vi "test_Series cRIO PWM TC Temp.vi"(8 "Error In":errorcluster) -> (0 "Error Out":errorcluster)   [LabVIEW 2023]
uses:
  DIO/DO DAQmx Fixed Freq PWM CFG/DO DAQmx Fixed Freq PWM CFG.lvclass
  Devices/NEO480HTA/Real All CFG/Read All CFG.lvclass
  Series/Series Base/Series Base.lvclass
  <vilib>/ActorFramework/Actor/Actor.lvclass
  <vilib>/ActorFramework/Stop Msg/Stop Msg.lvclass
  Sample Tasks/Sample Airtemp PWM Control/Sample Airtemp PWM Control.lvclass
  Thermometer/Virtual Thermometers/Virt Temperature Reader/Virt Temperature Reader.lvclass
  Series/Series Actor/Series Actor/Series Actor.lvclass
  Series/ISeries Actor/ISeries Actor Messages/Start Tasks Msg/Start Tasks Msg.lvclass
  Series/ISeries Actor/ISeries Actor Messages/Stop Tasks Msg/Stop Tasks Msg.lvclass
  DIO/Virtual DIO/Virt PWM Fixed Freq Generator/Virt DAQmx Fixed Freq PWM Generator.lvclass
panel:
  out "Aircooler Dutycycle":dbl=23.0
  in  "Start Series Button":bool
  in  "Kill Series Actor Button":bool
  out "Temperature Chart Lossy":dbl(graph)
  in  "Temp Setpoint":dbl=23.0 format="%#_g °C"
  in  "stop":bool
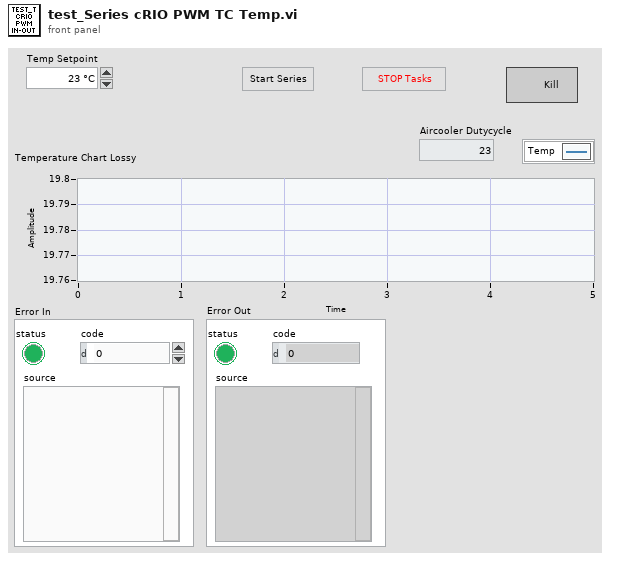
[diagram p1: front panel]
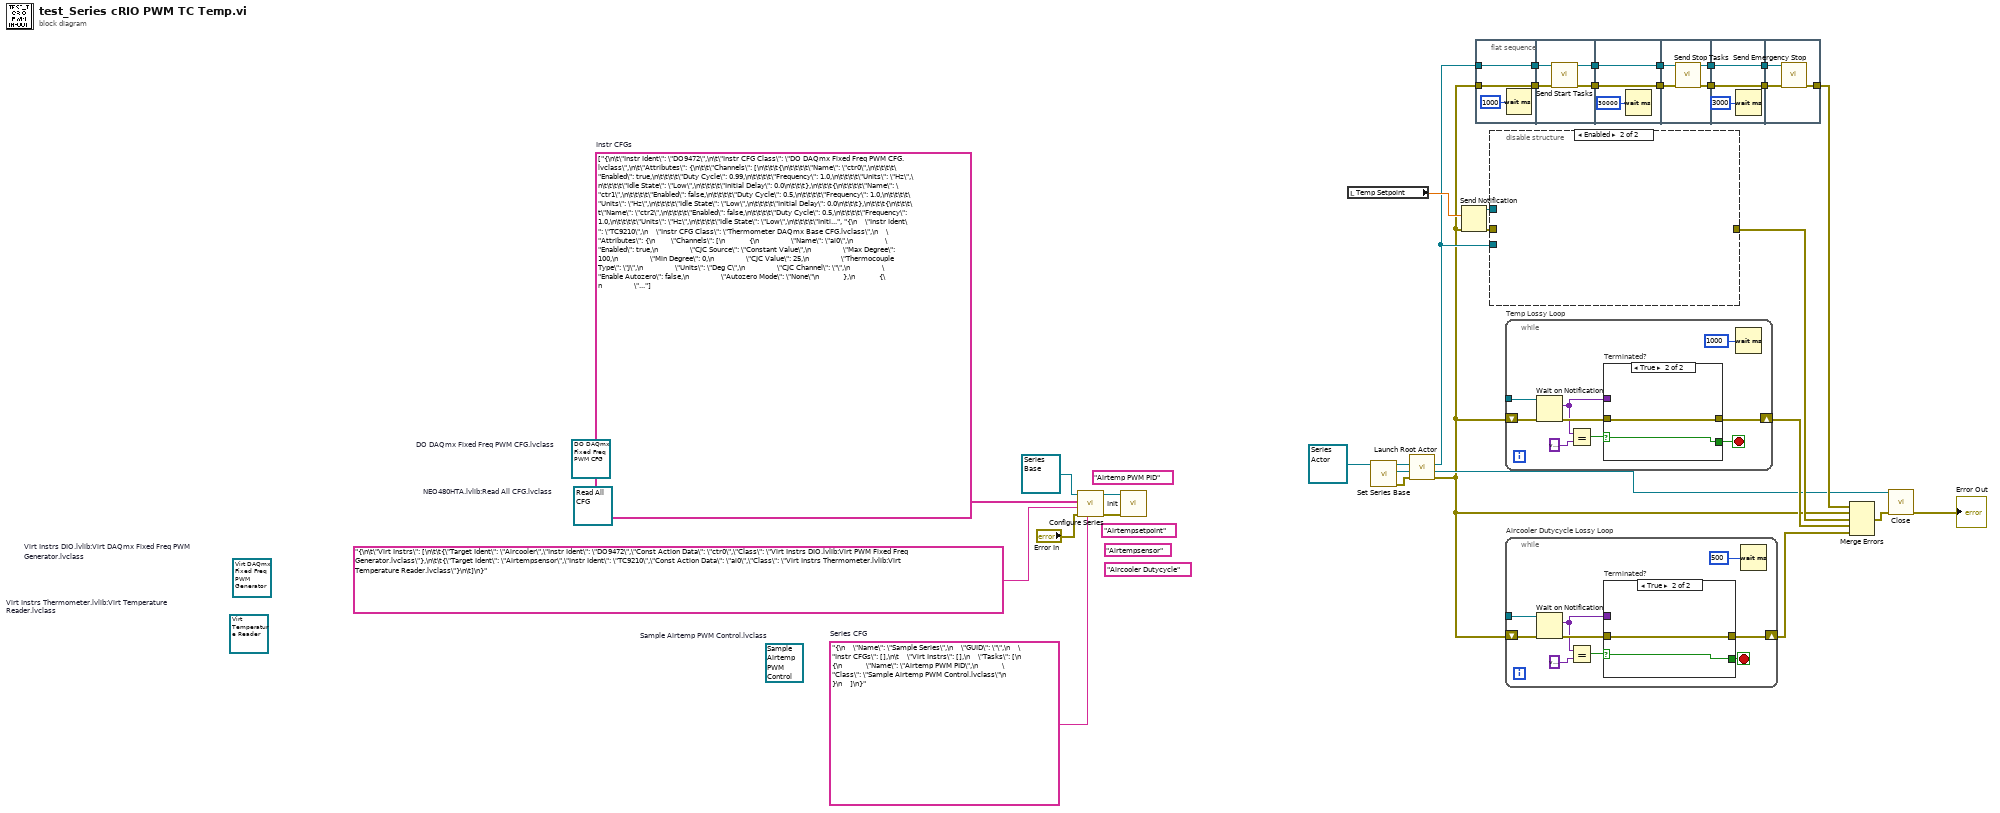
[diagram p0: block diagram]
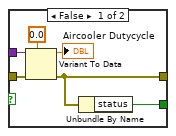
[diagram p2: hidden frame]
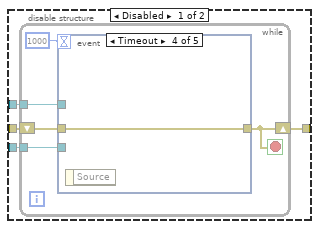
[diagram p3: hidden frame]
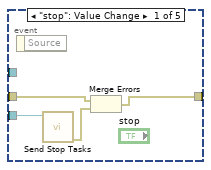
[diagram p4: hidden frame]
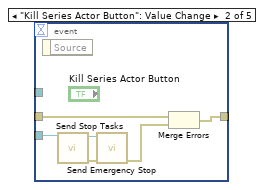
[diagram p5: hidden frame]
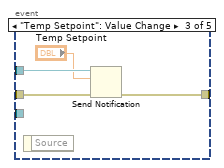
[diagram p6: hidden frame]
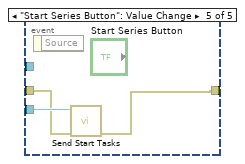
[diagram p7: hidden frame]
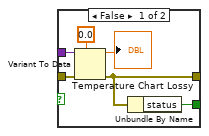
[diagram p8: hidden frame]
diagram:
  w4 = "Aircooler Dutycycle" ("Notifier Name")
  (unwired) refnum<class "Virt Temperature Reader.lvclass"> refnum  # Virt Instrs Thermometer.lvlib:Virt Temperature Reader.lvclass
  (unwired) refnum<class "Sample Airtemp PWM Control.lvclass"> refnum  # Sample Airtemp PWM Control.lvclass
  w26 = "Airtempsensor" ("Target Name")
  w5 = "Airtemp PWM PID"
  w28 = "Airtempsetpoint" ("Name")
  (unwired) refnum<class "Virt DAQmx Fixed Freq PWM Generator.lvclass"> refnum  # Virt Instrs DIO.lvlib:Virt DAQmx Fixed Freq PWM Generator.lvclass
  w39 = "{\n    \"Name\": \"Sample Series\",\n    \"GUID\": \"\",\n    \"Instr CFGs\": [],\n\t    \"Virt Instrs\": [],\n    \"Tasks\": [\n        {\n            \"Name\": \"Airtemp PWM PID\",\n            \"Class\": \"Sample Airtemp PWM Control.lvclass\"\n        }\n    ]\n}"  # Series CFG
  (unwired) refnum<class "Read All CFG.lvclass"> refnum  # NEO480HTA.lvlib:Read All CFG.lvclass
  (unwired) refnum<class "DO DAQmx Fixed Freq PWM CFG.lvclass"> refnum  # DO DAQmx Fixed Freq PWM CFG.lvclass
  w37 = string[] ["{\n\t\"Instr Ident\": \"DO9472\",\n\t\"Instr CFG Class\": \"DO DAQmx Fixed Freq PWM CFG.lvclass\",\n\t\"Attributes\": {\n\t\t\"Channels\": [\n\t\t\t{\n\t\t\t\t\"Name\": \"ctr0\",\n\t\t\t\t\"Enabled\": true,\n\t\t\t\t\"Duty Cycle\": 0.99,\n\t\t\t\t\"Frequency\": 1.0,\n\t\t\t\t\"Units\": \"Hz\",\n\t\t\t\t\"Idle State\": \"Low\",\n\t\t\t\t\"Initial Delay\": 0.0\n\t\t\t},\n\t\t\t{\n\t\t\t\t\"Name\": \"ctr1\",\n\t\t\t\t\"Enabled\": false,\n\t\t\t\t\"Duty Cycle\": 0.5,\n\t\t\t\t\"Frequency\": 1.0,\n\t\t\t\t\"Units\": \"Hz\",\n\t\t\t\t\"Idle State\": \"Low\",\n\t\t\t\t\"Initial Delay\": 0.0\n\t\t\t},\n\t\t\t{\n\t\t\t\t\"Name\": \"ctr2\",\n\t\t\t\t\"Enabled\": false,\n\t\t\t\t\"Duty Cycle\": 0.5,\n\t\t\t\t\"Frequency\": 1.0,\n\t\t\t\t\"Units\": \"Hz\",\n\t\t\t\t\"Idle State\": \"Low\",\n\t\t\t\t\"Initial Delay\": 0.0\n\t\t\t},\n\t\t\t{\n\t\t\t\t\"Name\": \"ctr3\",\n\t\t\t\t\"Enabled\": false,\n\t\t\t\t\"Duty Cycle\": 0.5,\n\t\t\t\t\"Frequency\": 1.0,\n\t\t\t\t\"Units\": \"Hz\",\n\t\t\t\t\"Idle State\": \"Low\",\n\t\t\t\t\"Initial Delay\": 0.0\n\t\t\t}\n\t\t],\n\t\t\"Timing\": {\n\t\t\t\"Samples per Channel\": 1000,\n\t\t\t\"Sample Mode\": \"Continuous Samples\",\n\t\t\t\"Sample Rate\": 0.0,\n\t\t\t\"Sample Clock Source\": \"Implicit\",\n\t\t\t\"Active Edge\": \"Rising\"\n\t\t},\n\t\t\"Trigger\": {\n\t\t\t\"Trigger Type\": \"No Trigger\"\n\t\t}\n\t}\n}", "{\n    \"Instr Ident\": \"TC9210\",\n    \"Instr CFG Class\": \"Thermometer DAQmx Base CFG.lvclass\",\n    \"Attributes\": {\n        \"Channels\": [\n            {\n                \"Name\": \"ai0\",\n                \"Enabled\": true,\n                \"CJC Source\": \"Constant Value\",\n                \"Max Degree\": 100,\n                \"Min Degree\": 0,\n                \"CJC Value\": 25,\n                \"Thermocouple Type\": \"J\",\n                \"Units\": \"Deg C\",\n                \"CJC Channel\": \"\",\n                \"Enable Autozero\": false,\n                \"Autozero Mode\": \"None\"\n            },\n            {\n                \"Name\": \"ai1\",\n                \"Enabled\": false,\n                \"CJC Source\": \"Constant Value\",\n                \"Max Degree\": 100,\n                \"Min Degree\": 0,\n                \"CJC Value\": 25,\n                \"Thermocouple Type\": \"J\",\n                \"Units\": \"Deg C\",\n                \"CJC Channel\": \"\",\n                \"Enable Autozero\": false,\n                \"Autozero Mode\": \"None\"\n            },\n            {\n                \"Name\": \"ai2\",\n                \"Enabled\": false,\n                \"CJC Source\": \"Constant Value\",\n                \"Max Degree\": 100,\n                \"Min Degree\": 0,\n                \"CJC Value\": 25,\n                \"Thermocouple Type\": \"J\",\n                \"Units\": \"Deg C\",\n                \"CJC Channel\": \"\",\n                \"Enable Autozero\": false,\n                \"Autozero Mode\": \"None\"\n            },\n            {\n                \"Name\": \"ai3\",\n                \"Enabled\": false,\n                \"CJC Source\": \"Constant Value\",\n                \"Max Degree\": 100,\n                \"Min Degree\": 0,\n                \"CJC Value\": 25,\n                \"Thermocouple Type\": \"J\",\n                \"Units\": \"Deg C\",\n                \"CJC Channel\": \"\",\n                \"Enable Autozero\": false,\n                \"Autozero Mode\": \"None\"\n            }\n        ],\n        \"Timing\": {\n            \"Samples per Channel\": 1000,\n            \"Sample Mode\": \"Continuous Samples\",\n            \"Sample Rate\": 14,\n            \"Sample Clock Source\": \"OnboardClock\",\n            \"Active Edge\": \"Rising\"\n        },\n        \"Trigger\": {\n            \"Trigger Type\": \"No Trigger\"\n        },\n        \"Acquisition\": {\n            \"Relative To\": \"Current Read Position\",\n            \"Overwrite\": \"Do Not Overwrite Unread Samples\",\n            \"Samples per Fetch\": -1,\n            \"Timeout\": 1\n        }\n    }\n}"]  # Instr CFGs
  n1 = call "Configure Series.vi"("Series CFG"=w39, "error in (no error)"="Error In", "Virt Instrs CFG"="{\n\t\"Virt Instrs\": [\n\t\t{\"Target Ident\": \"Aircooler\",\"Instr Ident\": \"DO9472\",\"Const Action Data\": \"ctr0\",\"Class\": \"Virt Instrs DIO.lvlib:Virt PWM Fixed Freq Generator.lvclass\"},\n\t\t{\"Target Ident\": \"Airtempsensor\",\"Instr Ident\": \"TC9210\",\"Const Action Data\": \"ai0\",\"Class\": \"Virt Instrs Thermometer.lvlib:Virt Temperature Reader.lvclass\"}\n\t]\n}", "Instr CFGs"=w37, "HAL GOOP4:Series Base in"=refnum<class "Series Base.lvclass"> refnum ("HAL GOOP4.lvlib:Study Base.lvclass")) -> ("error out"=w41:errorcluster, "HAL GOOP4:Series Base out"=w42:refnum<class "Series Base.lvclass">)  [unwired: 5 in]
  n2 = call-dynamic "Init.vi"("error in"=w41, "HAL GOOP4:Series Base in"=w42) -> ("error out"=w35:errorcluster, "HAL GOOP4:Series Base out"=w31:refnum<class "Series Base.lvclass">)  [unwired: 8 in]
  n3 = local read "Temp Setpoint"() -> (w32:dbl)
  n4 = call "Set Series Base.vi"("Series Actor in"=refnum<class "Series Actor.lvclass"> refnum ("HAL GOOP4.lvlib:Series Actor.lvlib:Series Actor.lvclass")) -> ("error out"=w30:errorcluster, "Series Actor out"=w29:refnum<class "Series Actor.lvclass">, "error in (no error)"=w7:errorcluster, "Series Base"=w6:refnum<class "Series Base.lvclass">)  [unwired: 7 in]
  n5 = call <vilib>:"Launch Root Actor.vi"("error in (no error)"=w30, "Actor"=w29) -> ("error out"=w2:errorcluster, "Actor's Enqueuer"=w19:refnum<class "Message Enqueuer.lvclass">)  [unwired: 8 in]
  n6 = Send Notification(notification=w32, error in (no error)=w2) -> (notifier=w24:refnum<notifier>, notifier out=w23:refnum<notifier>, error out=w33:errorcluster)
  n7 = flat-sequence {
    tunnel: w2 -> [w44]
    tunnel: w19 -> [w45]
    tunnel: [w45] -> w18
    tunnel: [w44] -> w17
    tunnel: w18 -> [w49]
    tunnel: w17 -> [w48]
    tunnel: [w47] -> w16
    tunnel: [w46] -> w15
    tunnel: w16 -> [w51]
    tunnel: w15 -> [w50]
    tunnel: [w51] -> w14
    tunnel: [w50] -> w13
    tunnel: w14 -> [w55]
    tunnel: w13 -> [w56]
    tunnel: [w54] -> w11
    tunnel: [w53] -> w9
    tunnel: [w58] -> w12
    tunnel: w11 -> [w58]
    tunnel: [w57] -> w10
    tunnel: w9 -> [w57]
    tunnel: w12 -> [w61]
    tunnel: w10 -> [w62]
    tunnel: [w60] -> w8
    frame #0 {
      n8 = Wait (ms)(milliseconds to wait=u32 1000) -> ()  [unwired: 1 out]
    }
    frame #1 {
      n9 = call "Send Start Tasks.vi"("error in (no error)"=w48, "Message Enqueuer"=w49) -> ("error out"=w46:errorcluster, "Message Enqueuer out"=w47:refnum<class "Message Enqueuer.lvclass">)  [unwired: 8 in]
    }
    frame #2 {
      n10 = Wait (ms)(milliseconds to wait=u32 30000) -> ()  [unwired: 1 out]
    }
    frame #3 {
      n11 = call "Send Stop Tasks.vi"("error in (no error)"=w56, "Message Enqueuer"=w55) -> ("error out"=w53:errorcluster, "Message Enqueuer out"=w54:refnum<class "Message Enqueuer.lvclass">)  [unwired: 8 in]
    }
    frame #4 {
      n12 = Wait (ms)(milliseconds to wait=u32 3000) -> ()  [unwired: 1 out]
    }
    frame #5 {
      n13 = call <vilib>:"Send Emergency Stop.vi"("error in (no error)"=w62, "Message Enqueuer"=w61) -> ("error out"=w60:errorcluster)  [unwired: 9 in]
    }
  }
  n14 = disable-structure shown="Enabled" {
    disable-tunnel: w33 -> [w66 _]
    disable-tunnel: w23 -> [w65 _]
    disable-tunnel: [w64 _] -> w20
    disable-tunnel: w19 -> [w63 _]
    frame Disabled {
      n15 = while {
        shift-right: [w71] -> w64
        shift-left: w66 -> [w70]
        tunnel: w63 -> [w69]
        tunnel: w65 -> [w68]
        stop <- w71 stop-if-true
        n16 = event shown="[3] Timeout" {
          selector: _ -> [_ _ _ _ _]
          dyn-events: _ -> [_ _ _ _ _]
          timeout: 1000 -> [_ _ _ _ _]
          tunnel: [w72 w79 w83 w86 w87] -> w71
          tunnel: w68 -> [_ _ w85 _ _]
          tunnel: w70 -> [w73 w78 w82 w86 w88]
          tunnel: w69 -> [w75 w81 _ _ w89]
          event "stop": Value Change {
            n17 = event-data() -> ()  [unwired: 1 in, 1 out]
            n18 = call "Send Stop Tasks.vi"("Message Enqueuer"=w75) -> ("error out"=w74:errorcluster)  [unwired: 9 in, 1 out]
            n19 = Merge Errors(w73, w74) -> (w72:errorcluster)
          }
          event "Kill Series Actor Button": Value Change {
            n20 = event-data() -> ()  [unwired: 1 in, 1 out]
            n21 = call "Send Stop Tasks.vi"("Message Enqueuer"=w81) -> ("error out"=w80:errorcluster, "Message Enqueuer out"=w76:refnum<class "Message Enqueuer.lvclass">)  [unwired: 9 in]
            n22 = call <vilib>:"Send Emergency Stop.vi"("error in (no error)"=w80, "Message Enqueuer"=w76) -> ("error out"=w77:errorcluster)  [unwired: 9 in]
            n23 = Merge Errors(w78, w77) -> (w79:errorcluster)
          }
          event "Temp Setpoint": Value Change {
            n24 = event-data() -> ()  [unwired: 1 in, 1 out]
            n25 = Send Notification(notification="Temp Setpoint", notifier=w85, error in (no error)=w82) -> (error out=w83:errorcluster)  [unwired: 1 out]
          }
          event Timeout {
            n26 = event-data() -> ()  [unwired: 1 in, 1 out]
          }
          event "Start Series Button": Value Change {
            n27 = event-data() -> ()  [unwired: 1 in, 1 out]
            n28 = call "Send Start Tasks.vi"("error in (no error)"=w88, "Message Enqueuer"=w89) -> ("error out"=w87:errorcluster)  [unwired: 8 in, 1 out]
          }
        }
      }
    }
    frame Enabled {
    }
  }
  n29 = while "Temp Lossy Loop" {
    tunnel: [w94] -> w25
    shift-right: [w95] -> w21
    shift-left: w2 -> [w96]
    stop <- w93 stop-if-true
    n30 = Wait on Notification(notifier=w94, error in (no error)=w96) -> (notification=w91:variant, error out=w98:errorcluster)  [unwired: 2 in, 2 out]
    n31 = Equal?(x=w91, y=variant) -> (x = y?=w90:bool)
    n32 = case "Terminated?" shown="True" w90 {
      selector: w90 -> [_ w106]
      tunnel: w98 -> [w104 w105]
      tunnel: [w102 w105] -> w95
      tunnel: [w99 w106] -> w93
      tunnel: w91 -> [w100 _]
      frame False {
        n33 = Variant To Data(error in=w104, type=0.0 ("Waveform"), Variant=w100) -> (data=→"Temperature Chart Lossy":dbl, error out=w102:errorcluster)
        n34 = Unbundle By Name(w102) -> ("status"=w99:bool)
      }
      frame True {
      }
    }
    n35 = Wait (ms)(milliseconds to wait=u32 1000) -> ()  [unwired: 1 out]
  }
  n36 = while "Aircooler Dutycycle Lossy Loop" {
    tunnel: [w111] -> w3
    shift-right: [w112] -> w1
    shift-left: w2 -> [w113]
    stop <- w110 stop-if-true
    n37 = Wait on Notification(notifier=w111, error in (no error)=w113) -> (notification=w108:variant, error out=w115:errorcluster)  [unwired: 2 in, 2 out]
    n38 = Equal?(x=w108, y=variant) -> (x = y?=w107:bool)
    n39 = case "Terminated?" shown="True" w107 {
      selector: w107 -> [_ w123]
      tunnel: w115 -> [w121 w122]
      tunnel: [w119 w122] -> w112
      tunnel: [w117 w123] -> w110
      tunnel: w108 -> [w118 _]
      frame False {
        n40 = Variant To Data(error in=w121, type=0.0 ("Waveform"), Variant=w118) -> (data=→"Aircooler Dutycycle":dbl, error out=w119:errorcluster)
        n41 = Unbundle By Name(w119) -> ("status"=w117:bool)
      }
      frame True {
      }
    }
    n42 = Wait (ms)(milliseconds to wait=u32 500) -> ()  [unwired: 1 out]
  }
  n43 = Merge Errors(w8, w2, w20, w21, w1) -> (w22:errorcluster)
  n44 = call-dynamic "Close.vi"("error in"=w22, "Series Base in"=w6) -> ("error out"=→"Error Out":errorcluster)  [unwired: 8 in, 1 out]
